vi "获取年月日.vi"() -> (1 "数字ascii数组":u8[](array[numeric]), 2 "日期/时间字符串":string)   [LabVIEW 2015]
doc: "获取当前时间 并把时间字符串转换为ASCII数值数组"
panel:
  out "时间字符串":string
  out "秒":string
  out "分":string
  out "时":string
  out "日":string
  out "月":string
  out "年":string
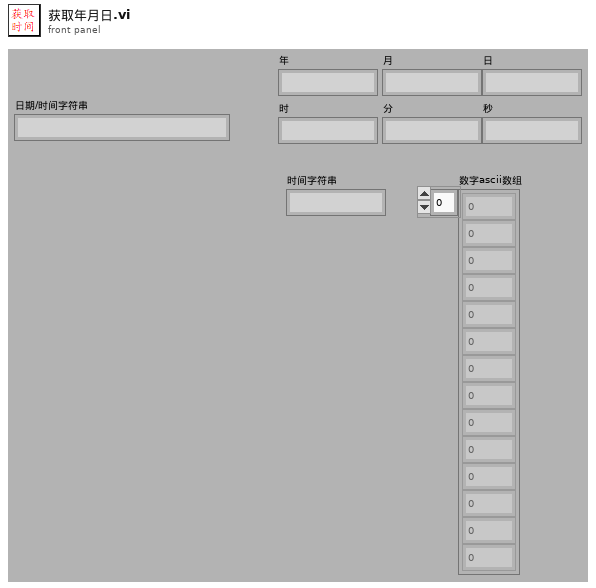
[diagram p1: front panel]
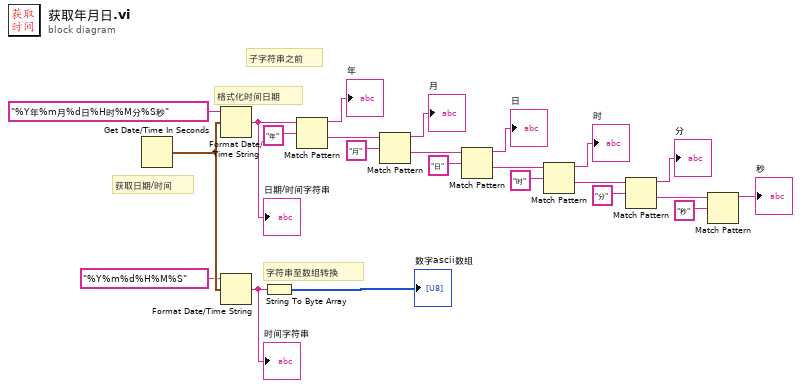
[diagram p0: block diagram]
diagram:
  # "字符串至数组转换"
  # "子字符串之前"
  # "格式化时间日期"
  # "获取日期/时间"
  n1 = Get Date/Time In Seconds() -> (seconds since 1Jan1904=w4:timestamp)
  n2 = Format Date/Time String(time format string (%c)="%Y年%m月%d日%H时%M分%S秒" ("时间格式字符串(%c)"), seconds (now)=w4) -> (date/time string=w22:string)  [unwired: 1 in]
  "日期/时间字符串" <- w22
  n3 = Format Date/Time String(time format string (%c)="%Y%m%d%H%M%S" ("时间格式字符串(%c)"), seconds (now)=w4) -> (date/time string=w2:string)  [unwired: 1 in]
  "时间字符串" <- w2
  n4 = String To Byte Array(string=w2) -> (unsigned byte array=→"数字ascii数组":u8[])
  n5 = Match Pattern(string=w22, regular expression="年" ("正则表达式")) -> (before substring=→"年":string, after substring=w10:string)  [unwired: 1 in, 2 out]
  n6 = Match Pattern(string=w10, regular expression="月" ("正则表达式")) -> (before substring=→"月":string, after substring=w9:string)  [unwired: 1 in, 2 out]
  n7 = Match Pattern(string=w9, regular expression="日" ("正则表达式")) -> (before substring=→"日":string, after substring=w8:string)  [unwired: 1 in, 2 out]
  n8 = Match Pattern(string=w8, regular expression="时" ("正则表达式")) -> (before substring=→"时":string, after substring=w7:string)  [unwired: 1 in, 2 out]
  n9 = Match Pattern(string=w7, regular expression="分" ("正则表达式")) -> (before substring=→"分":string, after substring=w6:string)  [unwired: 1 in, 2 out]
  n10 = Match Pattern(string=w6, regular expression="秒" ("正则表达式")) -> (before substring=→"秒":string)  [unwired: 1 in, 3 out]
